vi "refrence channel.vi"() -> ()   [LabVIEW 2020]
uses:
  <vilib>/Utility/error.llb/DialogType.ctl
  <vilib>/DAQmx/read.llb/DAQmx Read (Analog 1D Wfm NChan 1Samp).vi
  <vilib>/DAQmx/create/channels.llb/DAQmx Create Channel (AI-Voltage-Basic).vi
  <vilib>/DAQmx/miscellaneous.llb/DAQmx Fill In Error Info.vi
  <vilib>/DAQmx/configure/timing.llb/DAQmx Timing (Sample Clock).vi
  <resource>/objmgr/daqmx.rc
panel:
  out "Actual Sample Rate":dbl=1000.0 format="%0.2f"
  out "data 2":waveform(dbl)[](graph)
  out "Consumer Iteration 3":i32=1109257
  in  "stop 4":bool
  out "Producer Iteration 3":i32=1109256
  out "error out 3":errorcluster
  out "Loop Time (ms) 3":u32=10
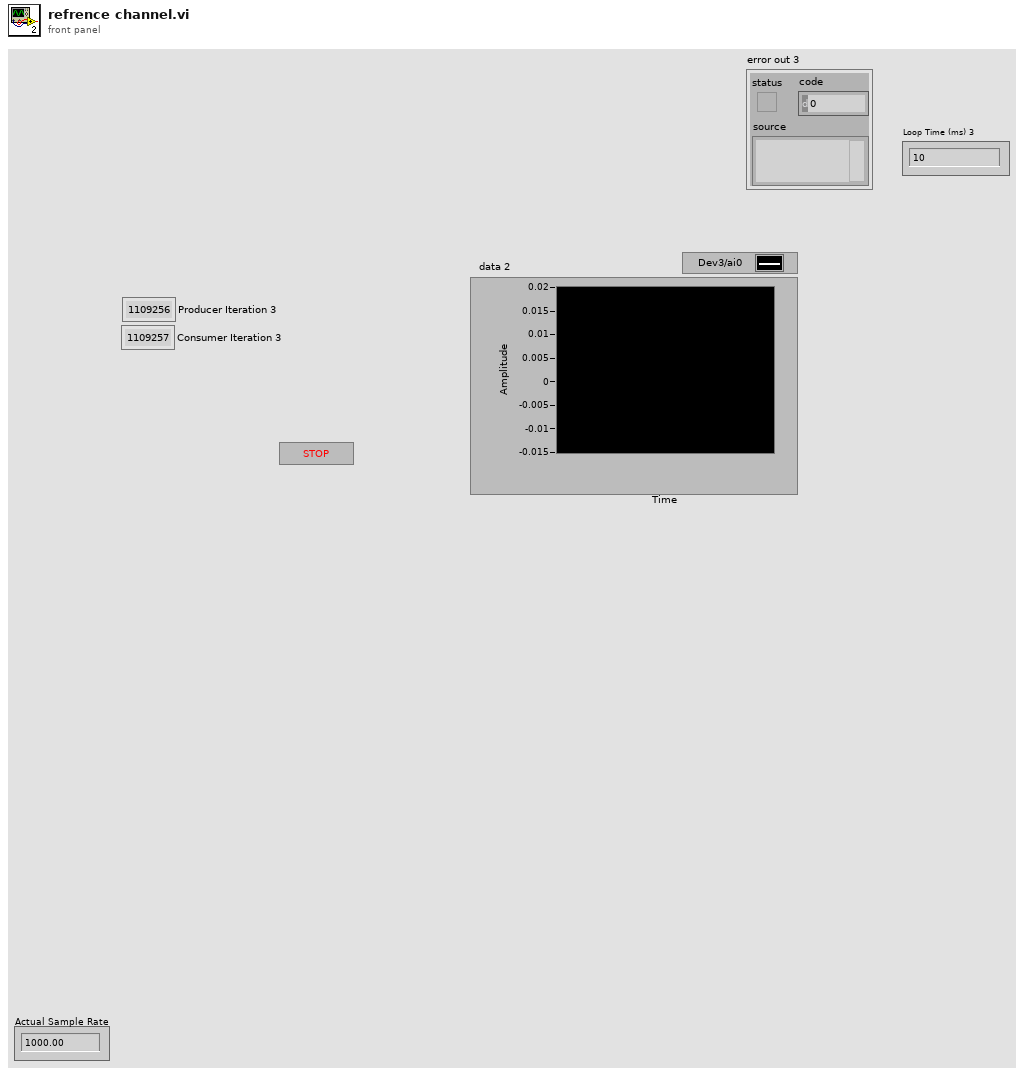
[diagram p1: front panel]
types:
  T1 = enum16{"open", "open or create", "create or replace", "create", "open (read-only)"}
  T2 = typedef "DialogType.ctl" = u16
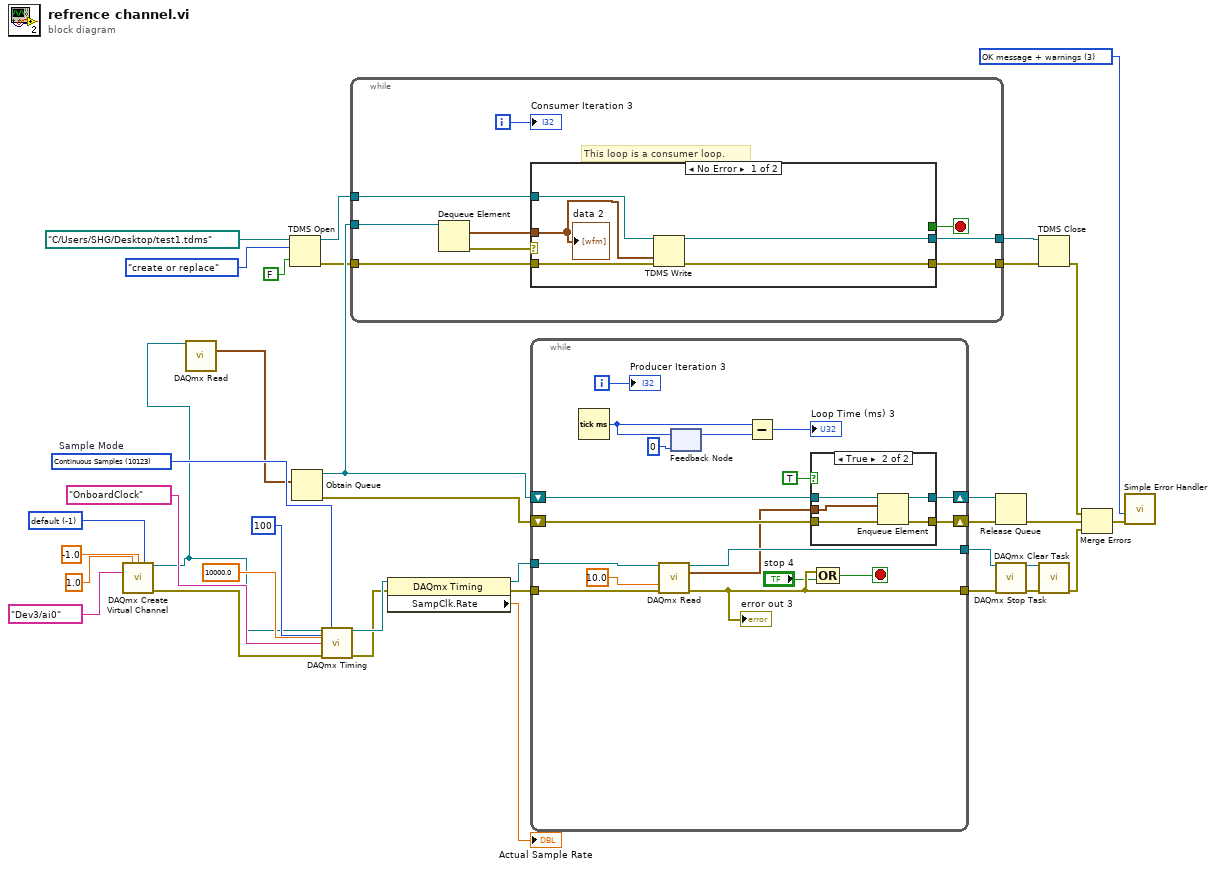
[diagram p0: block diagram]
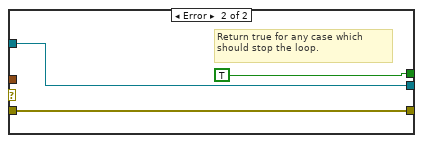
[diagram p2: hidden frame]
diagram:
  w6 = -1 items=["default"=-1, "RSE"=10083, "NRSE"=10078, "Differential"=10106, "Pseudodifferential"=12529] ("Terminal Configuration")
  w14 = 10123 items=["Finite Samples"=10178, "Continuous Samples"=10123, "Hardware Timed Single Point"=12522]  # Sample Mode
  w24 = T2 3 items=["no dialog", "OK message", "continue or stop message", "OK message + warnings", "continue/stop + warnings"] ("type of dialog (OK msg:1)")
  n1 = call-poly <vilib>:"DAQmx Create Virtual Channel.vi"("maximum value"=1.0 ("Max Voltage"), "minimum value"=-1.0 ("Min Voltage"), "input terminal configuration"=w6, "physical channels"=tag "Dev3/ai0" ("Physical Channel")) -> ("task out"=w1:refnum<k21>, "error out"=w13:errorcluster)  [unwired: 10 in]
  n2 = call-poly <vilib>:"DAQmx Read.vi"("task/channels in"=w1) -> ("data"=w2:waveform(dbl)[])  [unwired: 12 in, 2 out]
  n3 = TDMS Open(6:FALSE ("disable buffering? (T)"), 10:T1."create or replace" ("operation (0:open)"), 11:path "C:/Users/SHG/Desktop/test1.tdms" ("file path")) -> (0:w26:errorcluster, 3:w28:refnum<k34>)  [unwired: 4 in]
  n4 = Obtain Queue(element data type=w2) -> (queue out=w36:refnum<queue>, error out=w35:errorcluster)  [unwired: 4 in, 1 out]
  n5 = call-poly <vilib>:"DAQmx Timing.vi"("task/channels in"=w1, "sample mode"=w14, "samples per channel"=100 ("Number of Samples"), "rate"=10000.0 ("Sample Rate"), "source"=tag "OnboardClock" ("Sample Clock Source"), "error in"=w13) -> ("task out"=w16:refnum<k21>, "error out"=w15:errorcluster)  [unwired: 8 in]
  n6 = while {
    tunnel: w36 -> [w45]
    tunnel: w28 -> [w41]
    tunnel: [w40] -> w27
    tunnel: w26 -> [w39]
    tunnel: [w38] -> w25
    i -> [w42]
    stop <- w43 stop-if-true
    # "This loop is a consumer loop."
    n7 = Dequeue Element(queue=w45) -> (element=w37:waveform(dbl)[], error out=w44:errorcluster)  [unwired: 2 in, 2 out]
    n8 = case shown="No Error" w44 {
      tunnel: w37 -> [w46 _]
      tunnel: [_ TRUE] -> w43
      tunnel: w41 -> [w50 w52]
      tunnel: [w49 w52] -> w40
      tunnel: w39 -> [w48 w51]
      tunnel: [w47 w51] -> w38
      frame No Error {
        n9 = TDMS Write(0:w50, 9:w46, 11:w48) -> (4:w49:refnum<k34>, 15:w47:errorcluster)  [unwired: 3 in, 2 out]
        "data 2" <- w46
      }
      frame Error {
        # "Return true for any case which should stop the loop."
      }
    }
    "Consumer Iteration 3" <- w42
  }
  n10 = property class="DAQmx Timing"(reference=w16, error in=w15) -> (reference out=w11:refnum<k21>, error out=w10:errorcluster, "SampClk.Rate"=→"Actual Sample Rate":dbl)
  n11 = while {
    shift-right: [w62] -> w33
    shift-left: w35 -> [w69]
    shift-right: [w70] -> w34
    shift-left: w36 -> [w71]
    tunnel: [w67] -> w30
    tunnel: [w61] -> w29
    tunnel: w10 -> [w66]
    tunnel: w11 -> [w65]
    i -> [w63]
    stop <- w59 stop-if-true
    n12 = Tick Count (ms)() -> (millisecond timer value=w58:u32)
    n13 = call-poly <vilib>:"DAQmx Read.vi"("task/channels in"=w65, "timeout"=10.0, "error in"=w66) -> ("task out"=w67:refnum<k21>, "data"=w54:waveform(dbl)[], "error out"=w61:errorcluster)  [unwired: 10 in]
    "error out 3" <- w61
    n14 = feedback #1(u32 0 ("millisecond timer value")) -> (w57:u32)
    n15 = feedback-in #1(w58) -> ()
    n16 = Subtract(x=w58, y=w57) -> (x-y=→"Loop Time (ms) 3":u32)
    n17 = case shown="True" TRUE ("Case Constant\n(See Context Help)") {
      tunnel: w71 -> [w73 w78]
      tunnel: [w73 w77] -> w70
      tunnel: w69 -> [w72 w76]
      tunnel: [w72 w75] -> w62
      tunnel: w54 -> [_ w74]
      frame False {
      }
      frame True {
        n18 = Enqueue Element(queue=w78, element=w74, error in (no error)=w76) -> (queue out=w77:refnum<queue>, error out=w75:errorcluster)  [unwired: 1 in, 1 out]
      }
    }
    n19 = Compound Arithmetic op=OR(w61, "stop 4") -> (w59:bool)
    "Producer Iteration 3" <- w63
  }
  n20 = Release Queue(queue=w34, error in (no error)=w33) -> (error out=w19:errorcluster)  [unwired: 1 in, 2 out]
  n21 = call <vilib>:"DAQmx Stop Task.vi"("task/channels in"=w30, "error in"=w29) -> ("task out"=w31:refnum<k21>, "error out"=w32:errorcluster)  [unwired: 12 in]
  n22 = TDMS Close(8:w25, 11:w27) -> (0:w20:errorcluster)  [unwired: 1 out]
  n23 = call <vilib>:"DAQmx Clear Task.vi"("task in"=w31, "error in"=w32) -> ("error out"=w18:errorcluster)  [unwired: 13 in]
  n24 = Merge Errors(w20, w19, w18) -> (w23:errorcluster)
  n25 = call <vilib>:"Simple Error Handler.vi"("type of dialog (OK msg:1)"=w24, "error in (no error)"=w23) -> ()  [unwired: 3 in, 5 out]
